vi "PH_BL-Master.ShutterState 2 String.vi"(1 "Shutter State":T1) -> (0 "String":string)   [LabVIEW 2014, in "PH_BL-Master.lvlib"]
uses:
  PH_BL-Master.lvlib
  PH_BL-Master.Shutter State.ctl
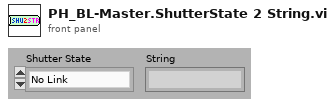
[diagram p1: front panel]
types:
  T1 = typedef "PH_BL-Master.lvlib/PH_BL-Master.Shutter State.ctl" = enum16{"No Link", "No Info", "In", "Out", "in between"}
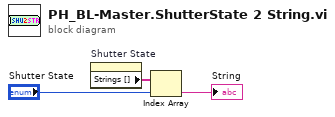
[diagram p0: block diagram]
diagram:
  n1 = property on="Shutter State" class="Enum (strict)"() -> ("Strings []"=w1:string[])  [unwired: 2 in, 2 out]
  n2 = Index Array(array=w1, index="Shutter State") -> (element=→"String":string)
